vi "Terminal-Utility-GetIPCDateTime.vi"(8 "error in (no error)":errorcluster caption="错误输入（无错误）") -> (0 "error out":errorcluster caption="错误输出", 3 "时间标识":timestamp)   [LabVIEW 2014]
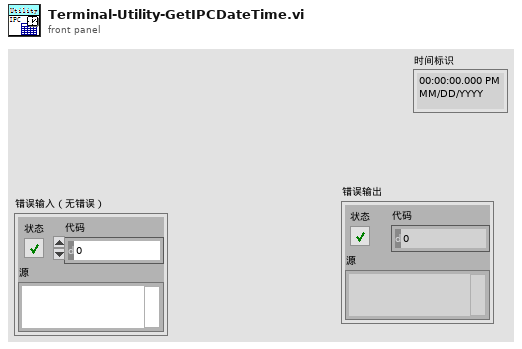
[diagram p1: front panel]
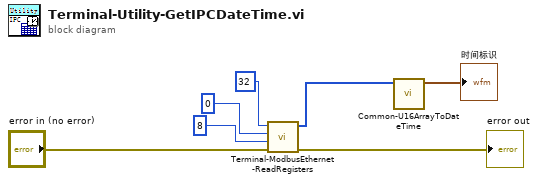
[diagram p0: block diagram]
diagram:
  n1 = call "Terminal-ModbusEthernet-ReadRegisters.vi"("error in"="error in (no error)", "number of holding registers"=u16 8, "starting address"=u16 0, "unit ID"=u8 32) -> ("error out"=→"error out":errorcluster, "register values"=w1:u16[])  [unwired: 6 in]
  n2 = call "Common-U16ArrayToDateTime.vi"("U16Array"=w1) -> ("时间标识"=→"时间标识":timestamp)  [unwired: 10 in]
